vi "disable Board.vi"(8 "error in (no error)":errorcluster, 9 "disable":bool, 10 "Board":u16, 11 "identifier":string) -> (0 "error out":errorcluster, 3 "function return":u32)   [LabVIEW 2015, in "XGL_DPP.lvlib"]
doc: "EXTERN DECLSPEC uint32_t CALL_CONV disableBoard(const char* identifier, uint16_t Board, bool disable);"
uses:
  XGL_DPP.lvlib
  XGL_DPP.dll
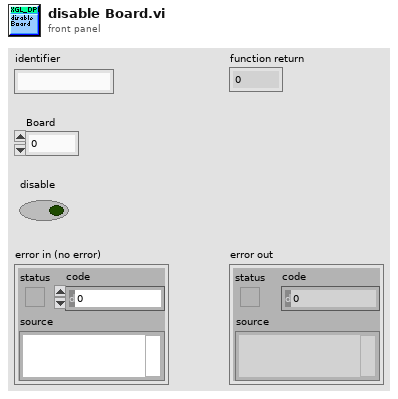
[diagram p1: front panel]
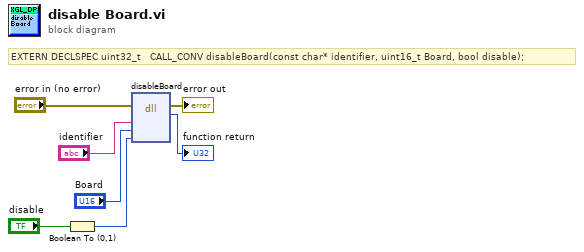
[diagram p0: block diagram]
diagram:
  # "EXTERN DECLSPEC uint32_t   CALL_CONV disableBoard(const char* identifier, uint16_t Board, bool disable);"
  n1 = Boolean To (0,1)(Boolean="disable") -> (0, 1=w3:i16)
  n2 = dll-call lib="D:/Users/XRF/Desktop/Scanning Software_Demokritos_2015_v7/libs/Vis_2/XGL_DPP.*" fn="disableBoard"(error in="error in (no error)", "identifier"="identifier", "Board"="Board", "disable"=w3) -> (error out=→"error out":errorcluster, →"function return":u32)  [unwired: 5 in, 1 out]
